vi "text encryption.vi"() -> ()   [LabVIEW 2022 SP3]
uses:
  <vilib>/Analysis/2dsp.llb/Real FFT.vi
  <vilib>/Analysis/NI_AALPro.lvlib
panel:
  out "text":string
  in  "read/write":enum16{"read/write", "read-only", "write-only"}(ring)
  in  "open or create":T1(ring)
  in  "Input file":path
  in  "Transmitting file":path
  out "Output":cdb[](array[numeric])
  out "FFT {X}":cdb[](array[numeric])
  out "ascii values":u8[](array[numeric])
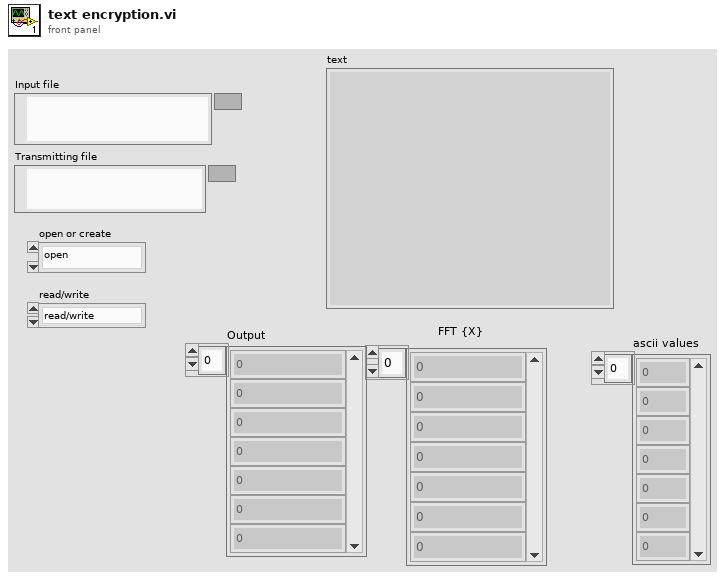
[diagram p1: front panel]
types:
  T1 = enum16{"open", "replace", "create", "open or create", "replace or create", "replace or create with confirmation"}
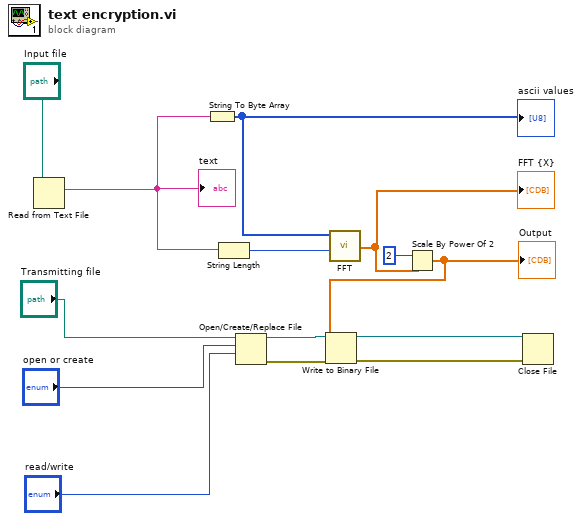
[diagram p0: block diagram]
diagram:
  n1 = Read from Text File(file (use dialog)="Input file") -> (text=w1:string)  [unwired: 3 in, 3 out]
  "text" <- w1
  n2 = String To Byte Array(string=w1) -> (unsigned byte array=w13:u8[])
  "ascii values" <- w13
  n3 = String Length(string=w1) -> (length=w14:i32)
  n4 = Open/Create/Replace File(file path (use dialog)="Transmitting file", operation (0:open)="open or create", access (0:read/write)="read/write") -> (refnum out=w10:refnum<file>, error out=w8:errorcluster)  [unwired: 3 in, 1 out]
  n5 = call-poly <vilib>:"FFT.vi"("FFT size"=w14, "X"=w13) -> ("FFT {X}"=w11:cdb[])  [unwired: 8 in, 1 out]
  "FFT {X}" <- w11
  n6 = Scale By Power Of 2(n=i16 2, x=w11) -> (x*2^n=w4:cdb[])
  "Output" <- w4
  n7 = Write to Binary File(file (use dialog)=w10, data=w4, error in=w8) -> (refnum out=w9:refnum<file>, error out=w7:errorcluster)  [unwired: 3 in, 1 out]
  n8 = Close File(refnum=w9, error in=w7) -> ()  [unwired: 2 out]
